vi "Correct_Position_infoY-15_TF.vi"() -> (0 "error out":errorcluster, 4 "Path":path)   [LabVIEW 2015]
panel:
  out "File Changed":bool
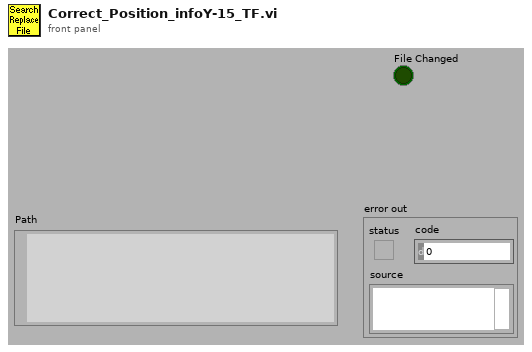
[diagram p1: front panel]
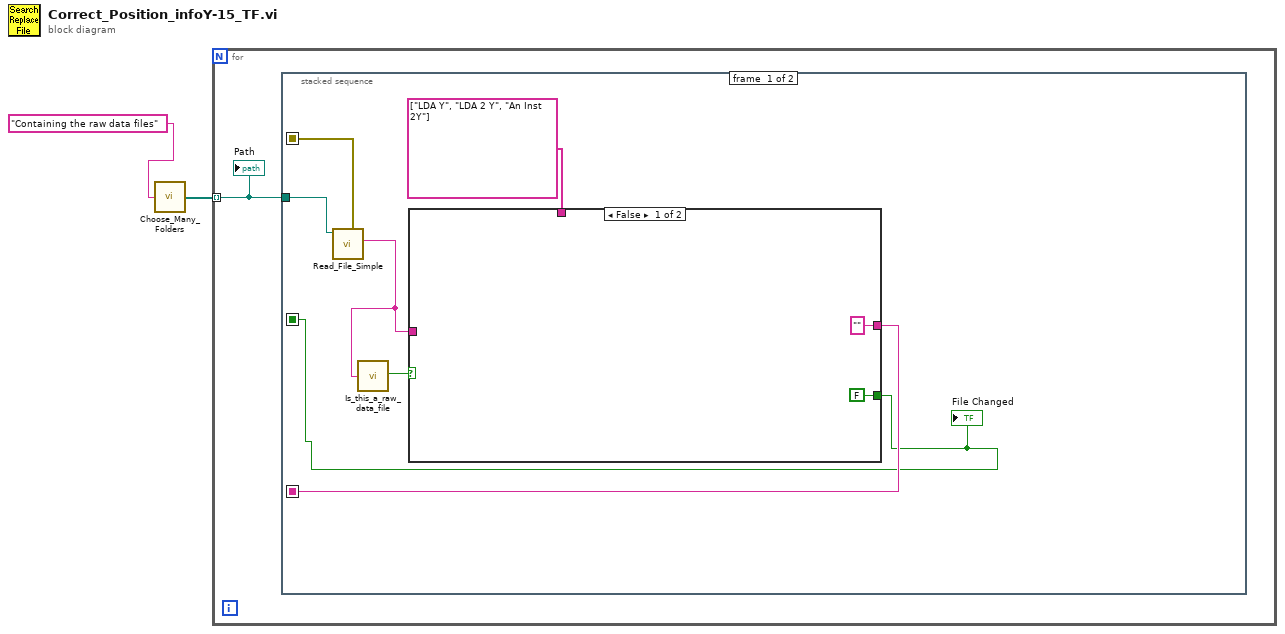
[diagram p0: block diagram]
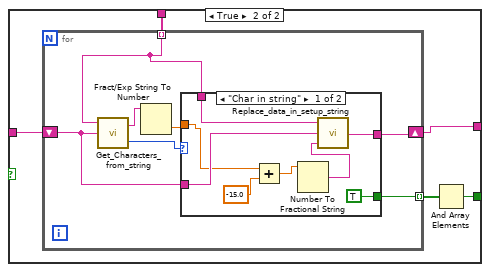
[diagram p2: hidden frame]
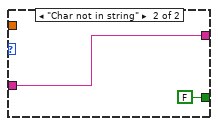
[diagram p3: hidden frame]
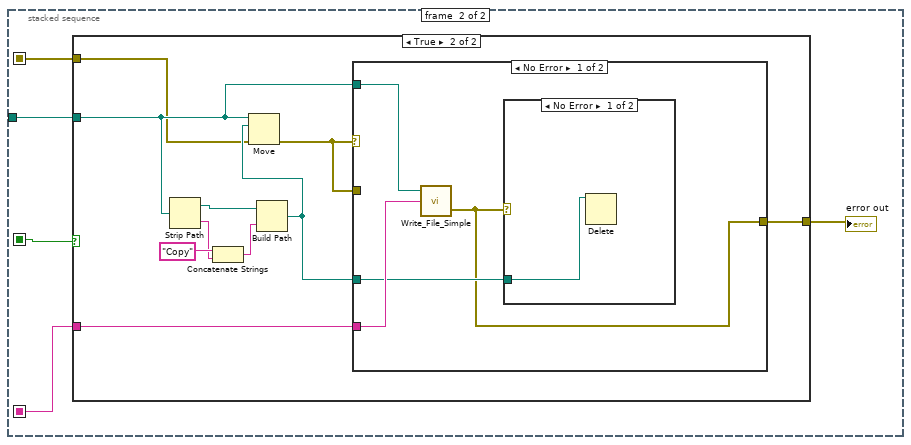
[diagram p4: hidden frame]
diagram:
  n1 = call "Choose_Many_Folders.vi"("Purpose of choosing folder"="Containing the raw data files") -> ("Files"=w1:path[])
  n2 = for {
    tunnel: w1 -> [w3] mode=indexing
    n3 = stacked-sequence {
      seq-local: [w9 _] -> [_ w35]
      seq-local: [w7 _] -> [_ w37]
      seq-local: [w6 _] -> [_ w36]
      tunnel: w3 -> [w10 w39]
      frame #0 {
        n4 = call "Read_File_Simple.vi"("Filename"=w10) -> ("error out"=w9:errorcluster, "string"=w4:string)  [unwired: 4 in, 4 out]
        n5 = call "Is_this_a_raw_data_file.vi"("character string"=w4) -> ("Raw Dat File?"=w5:bool)  [unwired: 2 out]
        n6 = case shown="False" w5 {
          tunnel: string[] ["LDA Y", "LDA 2 Y", "An Inst 2Y"] -> [_ w17]
          tunnel: ["" ("string") w16] -> w7
          tunnel: w4 -> [_ w15]
          tunnel: [FALSE w13] -> w6
          frame False {
          }
          frame True {
            n7 = for {
              shift-right: [w23] -> w16
              shift-left: w15 -> [w24]
              tunnel: w17 -> [w18] mode=indexing
              tunnel: [w21] -> w14 mode=indexing
              n8 = call "Get_Characters_from_string.vi"("Input string"=w24, "Variable name"=w18) -> ("Status"=w22:enum16{"Char in string", "Char not in string"}, "Value"=w20:string)  [unwired: 1 in]
              n9 = Fract/Exp String To Number(string=w20) -> (number=w19:dbl)  [unwired: 3 in, 1 out]
              n10 = case shown="\"Char in string\"" w22 {
                tunnel: w24 -> [w32 w34]
                tunnel: [w25 w34] -> w23
                tunnel: w19 -> [w29 _]
                tunnel: [TRUE FALSE] -> w21
                tunnel: w18 -> [w30 _]
                frame "Char in string" {
                  n11 = Add(x=w29, y=-15.0) -> (x+y=w27:dbl)
                  n12 = Number To Fractional String(number=w27) -> (F-format string=w26:string)  [unwired: 3 in]
                  n13 = call "Replace_data_in_setup_string.vi"("New data string"=w26, "Input string"=w32, "Variable name"=w30) -> ("Appended string"=w25:string)
                }
                frame "Char not in string" {
                }
              }
            }
            n14 = And Array Elements(Boolean array=w14) -> (logical AND=w13:bool)
          }
        }
        "File Changed" <- w6
      }
      frame #1 {
        n15 = case shown="True" w36 {
          tunnel: w39 -> [_ w46]
          tunnel: w37 -> [_ w45]
          tunnel: [w40 w43] -> w38
          tunnel: w35 -> [w40 w41]
          frame False {
          }
          frame True {
            n16 = Strip Path(path=w46) -> (stripped path=w47:path, name=w49:string)
            n17 = Concatenate Strings("Copy" ("name or relative path"), w49) -> (w48:string)
            n18 = Build Path(base path=w47, name or relative path=w48) -> (appended path=w44:path)
            n19 = Move(source path=w46, error in=w41, 10:w44) -> (error out=w42:errorcluster)  [unwired: 2 in, 2 out]
            n20 = case shown="No Error" w42 {
              tunnel: w46 -> [w54 _]
              tunnel: w45 -> [w53 _]
              tunnel: w44 -> [w52 _]
              tunnel: [w51 w56] -> w43
              tunnel: w42 -> [_ w56]
              frame No Error {
                n21 = call "Write_File_Simple.vi"("character string"=w53, "file path"=w54) -> ("error out"=w51:errorcluster)  [unwired: 1 in, 1 out]
                n22 = case shown="No Error" w51 {
                  tunnel: w52 -> [w55 _]
                  frame No Error {
                    n23 = Delete(path (use dialog)=w55) -> ()  [unwired: 4 in, 3 out]
                  }
                  frame Error {
                  }
                }
              }
              frame Error {
              }
            }
          }
        }
        "error out" <- w38
      }
    }
    "Path" <- w3
  }
